vi "about movie merge.vi"   [LabVIEW 2011]
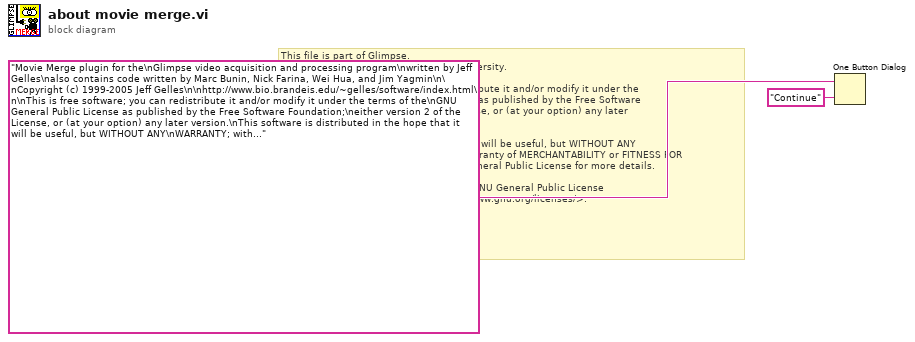
[diagram p0: block diagram]
diagram:
  # "This file is part of Glimpse. \nCopyright 2014 Jeff Gelles, Brandeis University.    \n\nGlimpse is free software: you can redistribute it and/or modify it under the \nterms of the GNU General Public License as published by the Free Software \nFoundation, either version 3 of the License, or (at your option) any later \nversion.\n\nGlimpse is distributed in the hope that it will be useful, but WITHOUT ANY \nWARRANTY; without even the implied warranty of MERCHANTABILITY or FITNESS FOR \nA PARTICULAR PURPOSE.  See the GNU General Public License for more details.\n\nYou should have received a copy of the GNU General Public License\nalong with Glimpse.  If not, see <http://www.gnu.org/licenses/>."
  n1 = One Button Dialog(message="Movie Merge plugin for the\nGlimpse video acquisition and processing program\nwritten by Jeff Gelles\nalso contains code written by Marc Bunin, Nick Farina, Wei Hua, and Jim Yagmin\n\nCopyright (c) 1999-2005 Jeff Gelles\n\nhttp://www.bio.brandeis.edu/~gelles/software/index.html\n\nThis is free software; you can redistribute it and/or modify it under the terms of the\nGNU General Public License as published by the Free Software Foundation;\neither version 2 of the License, or (at your option) any later version.\nThis software is distributed in the hope that it will be useful, but WITHOUT ANY\nWARRANTY; without even the implied warranty of MERCHANTABILITY or FITNESS\nFOR A PARTICULAR PURPOSE.  See the GNU General Public License for more details.\nYou should  receive a copy of the GNU General Public License along with each program;\nif not, write to the Free Software Foundation, Inc., 59 Temple Place, Suite 330,\nBoston, MA  02111-1307 USA. ", button name ("OK")="Continue") -> ()  [unwired: 1 out]
